vi "Compare Guess.vi"(10 "Guess":i32, 11 "Random Number":i32) -> (2 "Match?":bool, 3 "Guess Status":T1)   [LabVIEW 2013]
uses:
  controls/Guess Status.ctl
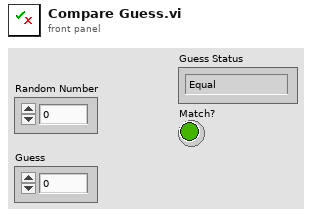
[diagram p1: front panel]
types:
  T1 = typedef "Guess Status.ctl" = enum16{"Equal", "Greater", "Less", "Error"}
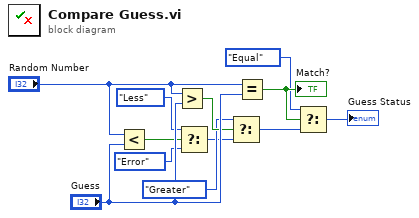
[diagram p0: block diagram]
diagram:
  n1 = Less?(x="Random Number", y="Guess") -> (x < y?=w2:bool)
  n2 = Greater?(x="Random Number", y="Guess") -> (0:w8:bool)
  n3 = Select(t=Guess_Status."Less", s=w2, f=Guess_Status."Error") -> (s? t:f=w5:T1)
  n4 = Select(t=Guess_Status."Greater", s=w8, f=w5) -> (s? t:f=w4:T1)
  n5 = Equal?(x="Random Number", y="Guess") -> (x = y?=w10:bool)
  "Match?" <- w10
  n6 = Select(t=Guess_Status."Equal", s=w10, f=w4) -> (s? t:f=→"Guess Status":T1)
